vi "niDTS WLAN INSTR TX.vi"(8 "error in (no error)":errorcluster, 9 "WLAN Tx Input Parameters":T2={"Standard"=enum."802.11 b DSSS", "DSSS Data Rate (Mbps)"=enum."1", "OFDM Data Rate (Mbps)"=enum."6", "MCS Index"=0, "N spatial streams"=0, "Chains"=[], "BandWidth (Hz)"=enum."20 MHz", "Channel"=0, "Gard Interval"=enum."LONG", "FEC Coding"=enum."BCC", "Dut Tx Power"=0.0, "16 symbols"=FALSE, "payload length bytes"=0, "idle interval"=0.0, "External Attenuation"=[], "Acquisition Parameters "={"Acquisition Length Mode"=enum."AUTO", "Acquisition Length (s)"=0.0, "Auto Level"=FALSE}, "TXP Measurement Parameters"={"TXP Power Enable"=FALSE, "TXP Averages"=0}, "ModAcc Measurement Paramaters"={"ModAcc Enable"=FALSE, "Header Detection"=enum."MANUAL", "Averages"=0, "Amplitude Tracking"=FALSE, "Channel Tracking"=FALSE, "Time Tracking"=FALSE, "Phase Tracking"=enum."NONE", "Clock Offset Est"=FALSE, "Impairments Est"=FALSE, "CFO Estimation"=enum."PAMBLE"}, "ModAcc DSSS Paramaters"={"DC Offset Compensation"=TRUE, "Equalization"=FALSE, "Phase Tracking"=TRUE, "Chip Start Location"=0, "Max Chips Used"=16, "Pulse Shaping FilterType"=enum."GAUSSIAN", "Pulse Shaping Filter Coefficient"=0.35}, "SEM Measurement Parameters"={"SEM Enable"=FALSE, "SEM Averages"=0, "Auto Span Enable"=FALSE, "Frequency Span (Hz)"=0.0, "Measurement Type"=enum."Standard", "Mask Frequencies (Hz)"=[], "Mask Power Offsets (dB)"=[]}, "OBW Measurement Parameters"={"OBW Enable"=FALSE, "OBW Averages"=0}, "DSSS Power Ramp"={"Power Ramp Enable"=FALSE, "Averages"=3, "Thresholds"={"Up Low (%)"=10.0, "Down Low (%)"=10.0, "Up High (%)"=90.0, "Down High (%)"=90.0}}, "Enable Traces"=FALSE} {"DSSS Power Ramp"."Thresholds"."Down High (%)" min=0.0 max=100.0 step=1.0; "DSSS Power Ramp"."Thresholds"."Up High (%)" min=0.0 max=100.0 step=1.0; "DSSS Power Ramp"."Thresholds"."Down Low (%)" min=0.0 max=100.0 step=1.0; "DSSS Power Ramp"."Thresholds"."Up Low (%)" min=0.0 max=100.0 step=1.0; "Acquisition Parameters"."Acquisition Length (s)" format="%#_6p"; "SEM Measurement Parameters"."Frequency Span (Hz)" format="%#_6p"; "idle interval" format="%_3p"}, 10 "RfsaWlan Handle":T1) -> (0 "error out":errorcluster, 3 "niDTS WLAN INSTR TX":refnum<class "niDTS WLAN INSTR TX.lvclass">)   [LabVIEW 2015, in "niDTS WLAN.lvlib" / "niDTS WLAN INSTR TX.lvclass"]
uses:
  niDTS WLAN INSTR TX.lvclass
  Tests/Tx Test/Includes/niDTS WLAN Tx Test INC Parameters.ctl
  Includes/niDTS WLAN INC Standard.ctl
  Includes/niDTS WLAN INC DSSS Data Rate.ctl
  Includes/niDTS WLAN INC OFDM Data Rate.ctl
  Includes/niDTS WLAN INC CH BW.ctl
  Includes/niDTS WLAN INC GI.ctl
  Includes/niDTS WLAN INC FEC Coding.ctl
  Includes/niDTS WLAN DUT INC Acquisition Parameters.ctl
  Includes/niDTS WLAN INC TXP Measurement Parameters.ctl
  Includes/niDTS WLAN INC ModAcc Measurement Parameters.ctl
  Includes/niDTS WLAN INC DSSS ModAcc Measurement Parameters.ctl
  Includes/niDTS WLAN INC Pulse Shaping Filter Type.ctl
  Includes/niDTS WLAN INC SEM Measurement Parameters.ctl
  Includes/niDTS WLAN INC OBW Measurement Parameters.ctl
  Includes/niDTS WLAN INC DSSS Power Ramp Parameters.ctl
  RiviInstDriver/niRfsaWlan/Includes/niRfsaWlan INC Handle.ctl
  RiviInstDriver/niRfsaWlan/Objects/niRfsaWlan.lvclass
  niDTS WLAN INSTR TX.lvclass/niDTS WLAN INSTR TX.ctl
  niDTS WLAN.lvlib
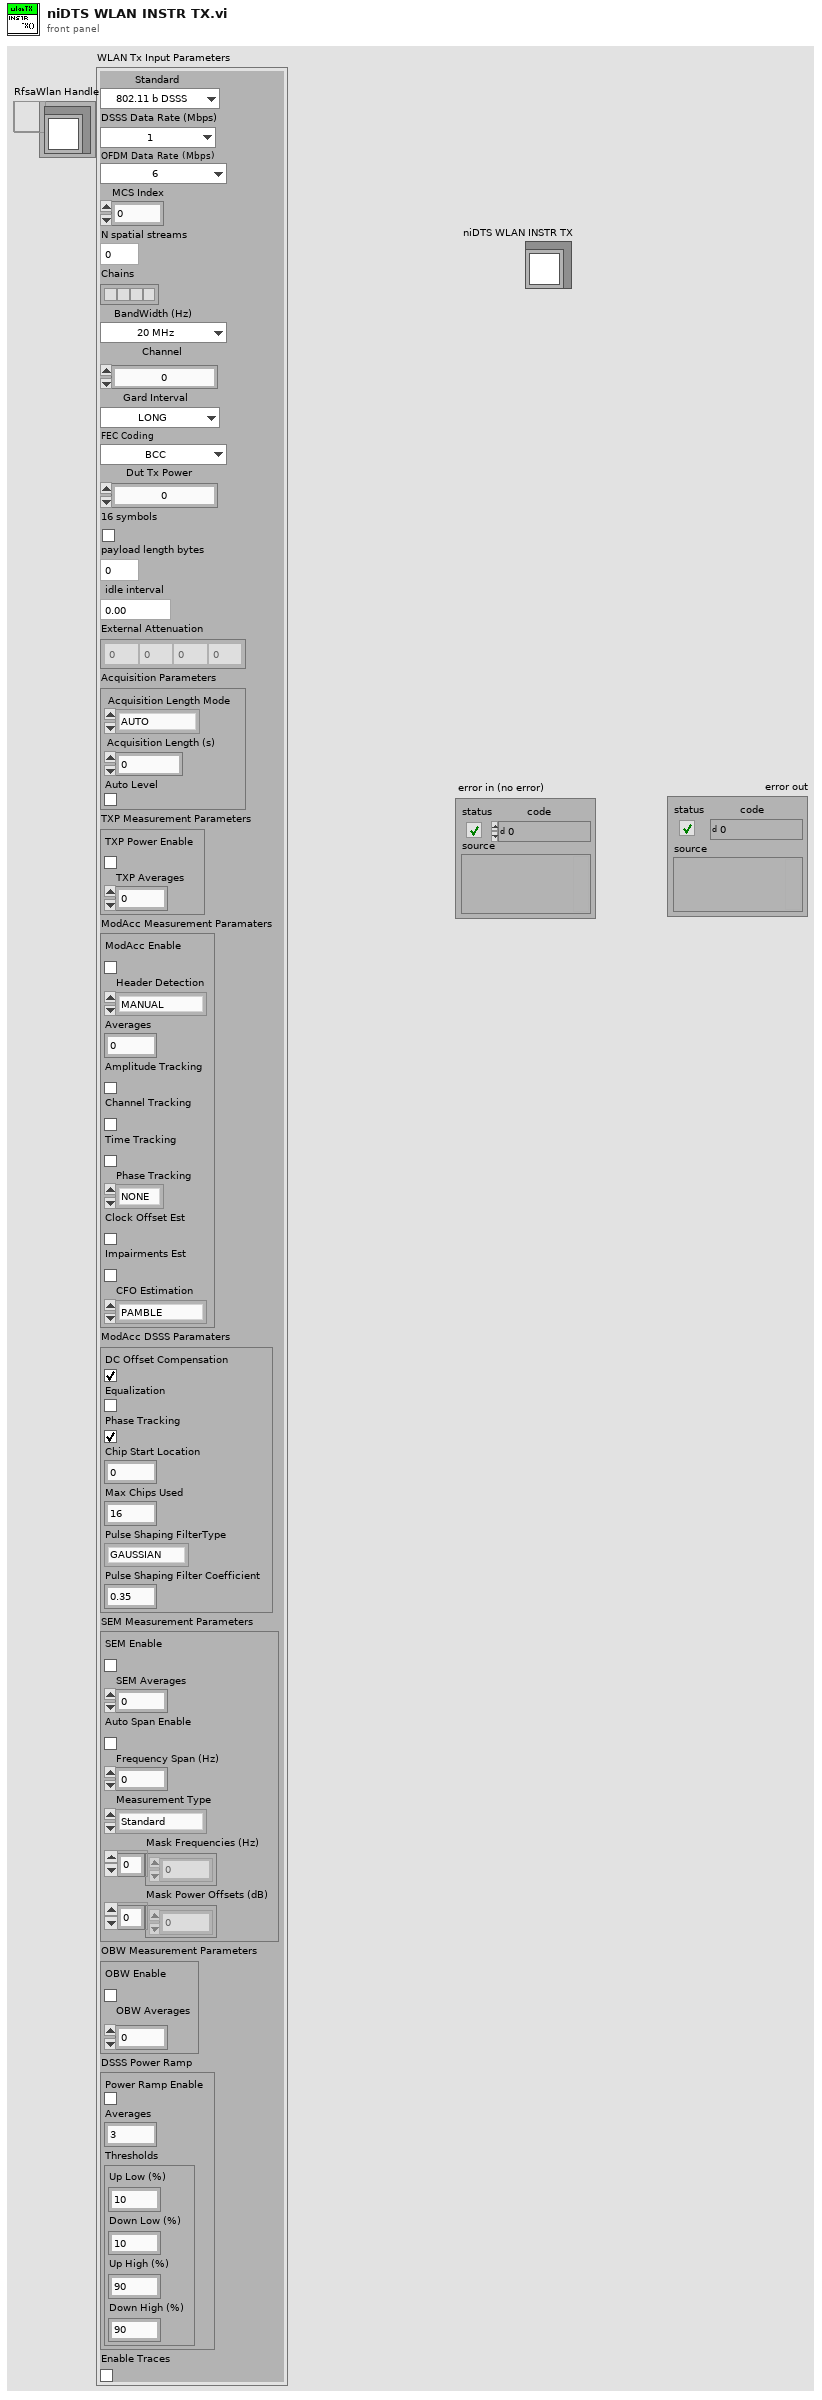
[diagram p1: front panel]
types:
  T1 = typedef "niRfsaWlan.lvclass/niRfsaWlan INC Handle.ctl" = refnum<data-value>
  T2 = typedef "niDTS WLAN.lvlib/niDTS WLAN Tx Test INC Parameters.ctl" = cluster{"Standard":T3, "DSSS Data Rate (Mbps)":T4, "OFDM Data Rate (Mbps)":T5, "MCS Index":i32, "N spatial streams":i32, "Chains":bool[], "BandWidth (Hz)":T6, "Channel":i32, "Gard Interval":T7, "FEC Coding":T8, "Dut Tx Power":dbl, "16 symbols":bool, "payload length bytes":i32, "idle interval":dbl, "External Attenuation":dbl[], "Acquisition Parameters ":T9, "TXP Measurement Parameters":T10, "ModAcc Measurement Paramaters":T11, "ModAcc DSSS Paramaters":T12, "SEM Measurement Parameters":T14, "OBW Measurement Parameters":T15, "DSSS Power Ramp":T16, "Enable Traces":bool}
  T3 = typedef "niDTS WLAN.lvlib/niDTS WLAN INC Standard.ctl" = enum16{"802.11 b DSSS", "802.11 a/g OFDM", "802.11 n HT", "802.11 ac VHT"}
  T4 = typedef "niDTS WLAN.lvlib/niDTS WLAN INC DSSS Data Rate.ctl" = enum16{"1", "2", "5.5", "11"}
  T5 = typedef "niDTS WLAN.lvlib/niDTS WLAN INC OFDM Data Rate.ctl" = enum16{"6", "9", "12", "18", "24", "36", "48", "54"}
  T6 = typedef "niDTS WLAN.lvlib/niDTS WLAN INC CH BW.ctl" = enum16{"20 MHz", "40 MHz", "80 MHz", "160 MHz"}
  T7 = typedef "niDTS WLAN.lvlib/niDTS WLAN INC GI.ctl" = enum16{"LONG", "SHORT"}
  T8 = typedef "niDTS WLAN.lvlib/niDTS WLAN INC FEC Coding.ctl" = enum16{"BCC", "LDPC"}
  T9 = typedef "niDTS WLAN.lvlib/niDTS WLAN DUT INC Acquisition Parameters.ctl" = cluster{"Acquisition Length Mode":enum16{"AUTO", "MANUAL"}, "Acquisition Length (s)":dbl, "Auto Level":bool}
  T10 = typedef "niDTS WLAN.lvlib/niDTS WLAN INC TXP Measurement Parameters.ctl" = cluster{"TXP Power Enable":bool, "TXP Averages":i32}
  T11 = typedef "niDTS WLAN.lvlib/niDTS WLAN INC ModAcc Measurement Parameters.ctl" = cluster{"ModAcc Enable":bool, "Header Detection":enum16{"MANUAL", "FIRST", "ALL"}, "Averages":i32, "Amplitude Tracking":bool, "Channel Tracking":bool, "Time Tracking":bool, "Phase Tracking":enum16{"NONE", "STANDARD", "CSF", "INSTANT"}, "Clock Offset Est":bool, "Impairments Est":bool, "CFO Estimation":enum16{"PAMBLE", "PDATA"}}
  T12 = typedef "niDTS WLAN.lvlib/niDTS WLAN INC DSSS ModAcc Measurement Parameters.ctl" = cluster{"DC Offset Compensation":bool, "Equalization":bool, "Phase Tracking":bool, "Chip Start Location":i16, "Max Chips Used":i16, "Pulse Shaping FilterType":T13, "Pulse Shaping Filter Coefficient":dbl}
  T13 = typedef "niDTS WLAN.lvlib/niDTS WLAN INC Pulse Shaping Filter Type.ctl" = enum16{"NONE", "RCOSINE", "RRCOSINE", "GAUSSIAN"}
  T14 = typedef "niDTS WLAN.lvlib/niDTS WLAN INC SEM Measurement Parameters.ctl" = cluster{"SEM Enable":bool, "SEM Averages":i32, "Auto Span Enable":bool, "Frequency Span (Hz)":dbl, "Measurement Type":enum16{"Standard", "Legacy", "Custom"}, "Mask Frequencies (Hz)":dbl[], "Mask Power Offsets (dB)":dbl[]}
  T15 = typedef "niDTS WLAN.lvlib/niDTS WLAN INC OBW Measurement Parameters.ctl" = cluster{"OBW Enable":bool, "OBW Averages":i32}
  T16 = typedef "niDTS WLAN.lvlib/niDTS WLAN INC DSSS Power Ramp Parameters.ctl" = cluster{"Power Ramp Enable":bool, "Averages":i32, "Thresholds":cluster{"Up Low (%)":dbl, "Down Low (%)":dbl, "Up High (%)":dbl, "Down High (%)":dbl}}
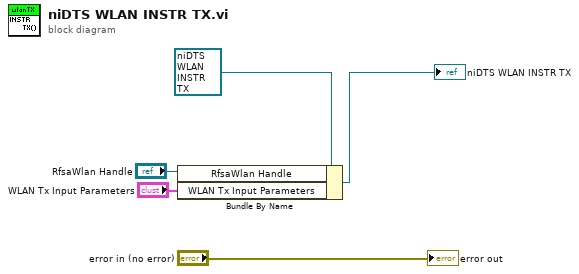
[diagram p0: block diagram]
diagram:
  n1 = Bundle By Name(cluster=refnum<class "niDTS WLAN INSTR TX.lvclass"> refnum ("niDTS WLAN.lvlib:niDTS WLAN INSTR TX"), "RfsaWlan Handle"="RfsaWlan Handle", "WLAN Tx Input Parameters"="WLAN Tx Input Parameters") -> (→"niDTS WLAN INSTR TX":refnum<class "niDTS WLAN INSTR TX.lvclass">)
  "error out" <- "error in (no error)"
